vi "Test Pixy2 Functionality.vi"() -> ()   [LabVIEW 2018]
uses:
  source/library/Types/Intersection.ctl
  source/library/Types/Vector.ctl
  <vilib>/Rock Robotics/WPI/SerialPort/WPI_SerialPort.ctl
  source/library/Interface/Pixy Com.lvclass
  source/deviceSupport/FRC/I2C/RoboRIO I2C.lvclass
  <vilib>/Rock Robotics/SystemInterfaces/i2clib/i2c_bus.ctl
  source/library/Pixy2.lvlib
  <vilib>/Rock Robotics/SystemInterfaces/spilib/spi_bus.ctl
  source/deviceSupport/FRC/SPI/RoboRIO SPI.lvclass
  source/deviceSupport/FRC/UART/RoboRIO UART.lvclass
panel:
  out "vectors":T1[](array[typedef])
  out "intersections":T2[](array[typedef])
  out "view":picture
  in  "Stop Button":bool
  in  "message":enum32{"RGB", "Lamp", "Blocks", "Lines"}(tab)
  in  "color":cluster{"r":u8, "g":u8, "b":u8}
  in  "lamp enable":cluster{"upper":bool, "lower":bool}
  in  "signature map":u8=255 format="%.0x"
  in  "max blocks":u8=255
  in  "features":enum16{"Main Features", "All Features"}(ring)
  in  "feature map":u8=7 format="%.0x"
  out "error out":errorcluster
  in  "send":bool
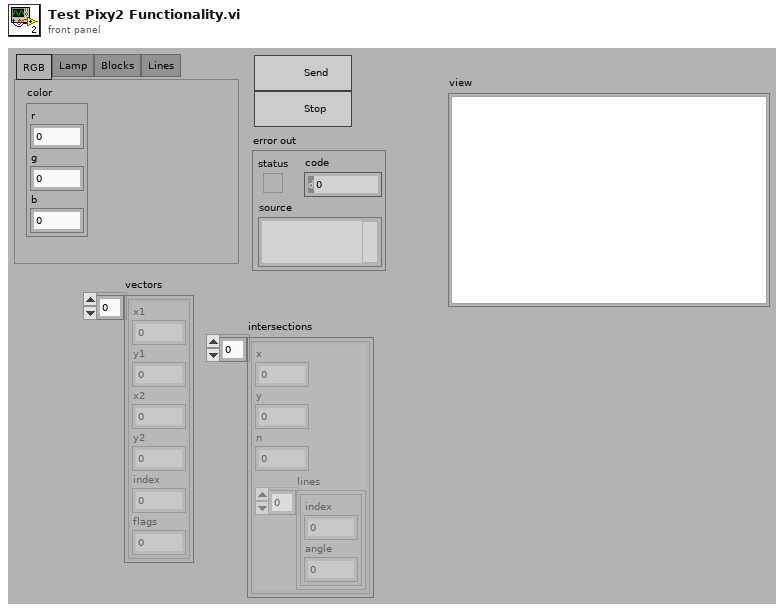
[diagram p1: front panel]
types:
  T1 = typedef "Pixy2.lvlib/Vector.ctl" = cluster{"x1":u8, "y1":u8, "x2":u8, "y2":u8, "index":u8, "flags":u8}
  T2 = typedef "Pixy2.lvlib/Intersection.ctl" = cluster{"x":u8, "y":u8, "n":u8, "lines":cluster{"index":u8, "angle":i16}[]}
  T3 = typedef "i2c_bus.ctl" = enum16{"I2C On-Board", "I2C MXP", "Invalid"}
  T4 = typedef "spi_bus.ctl" = enum16{"SPI On-Board, CS0", "SPI On-Board, CS1", "SPI On-Board, CS2", "SPI On-Board, CS3", "SPI MXP", "Invalid"}
  T5 = typedef "WPI_SerialPort.ctl" = enum16{"Onboard RS-232", "MXP TTL", "USB 1", "USB 2"}
  T6 = typedef "Pixy2.lvlib/Block.ctl" = cluster{"signature":u16, "x":u16, "y":u16, "width":u16, "height":u16, "angle":i16, "index":u8, "age":u8}
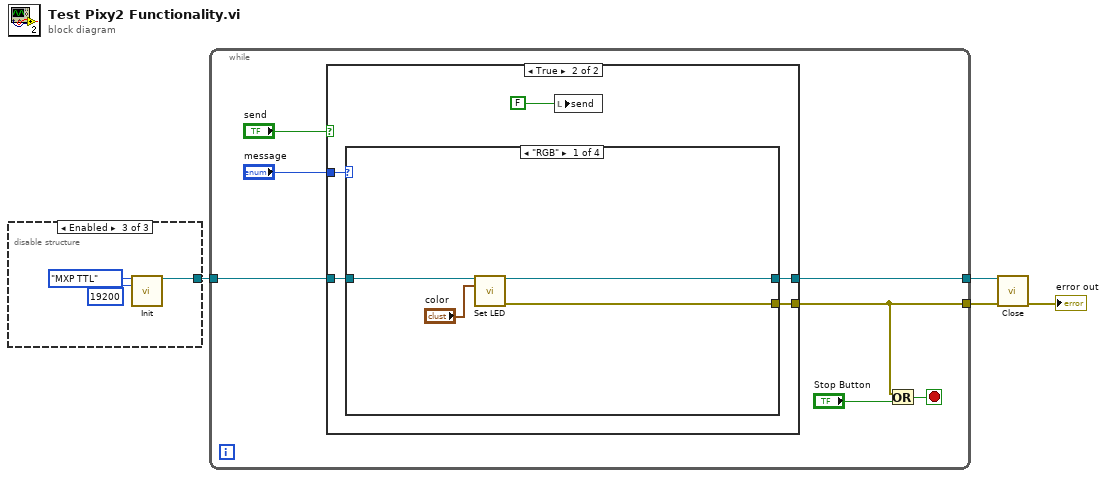
[diagram p0: block diagram]
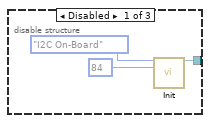
[diagram p2: hidden frame]
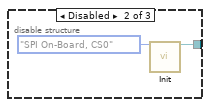
[diagram p3: hidden frame]
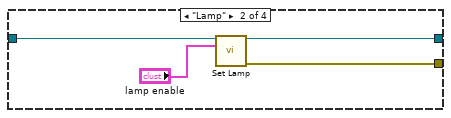
[diagram p5: hidden frame]
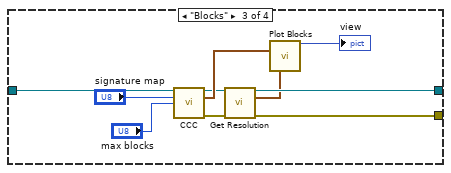
[diagram p6: hidden frame]
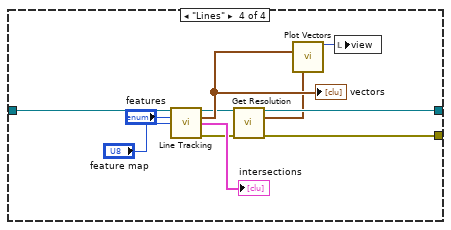
[diagram p7: hidden frame]
diagram:
  n1 = disable-structure shown="Enabled" {
    disable-tunnel: [w7 w9 w12] -> w4
    frame Disabled {
      n2 = call "Init.vi"("I2C Bus"=i2c_bus."I2C On-Board", "Device Address"=u8 84) -> ("comm interface out"=w7:refnum<class "Pixy Com.lvclass">)  [unwired: 12 in, 1 out]
    }
    frame Disabled {
      n3 = call "Init.vi"("SPI Bus"=spi_bus."SPI On-Board, CS0") -> ("comm interface out"=w9:refnum<class "Pixy Com.lvclass">)  [unwired: 13 in, 1 out]
    }
    frame Enabled {
      n4 = call "Init.vi"("serial port"=WPI_SerialPort."MXP TTL", "baud rate"=u32 19200) -> ("comm interface out"=w12:refnum<class "Pixy Com.lvclass">)  [unwired: 12 in, 1 out]
    }
  }
  n5 = while {
    tunnel: w4 -> [w18]
    tunnel: [w16] -> w3
    tunnel: [w17] -> w2
    stop <- w15 stop-if-true
    n6 = case shown="True" "send" {
      tunnel: w18 -> [w20 w24]
      tunnel: [_ w22] -> w16
      tunnel: [w20 w23] -> w17
      tunnel: "message" -> [_ w21]
      frame False {
      }
      frame True {
        n7 = case shown="\"RGB\"" w21 {
          tunnel: w24 -> [w29 w33 w43 w54]
          tunnel: [w28 w32 w35 w46] -> w23
          tunnel: [w27 w30 w36 w45] -> w22
          frame "RGB" {
            n8 = call "Set LED.vi"("comm interface in"=w29, "color"="color") -> ("comm interface out"=w28:refnum<class "Pixy Com.lvclass">, "error out"=w27:errorcluster)  [unwired: 12 in]
          }
          frame "Lamp" {
            n9 = call "Set Lamp.vi"("comm interface in"=w33, "lamp enable"="lamp enable") -> ("comm interface out"=w32:refnum<class "Pixy Com.lvclass">, "error out"=w30:errorcluster)  [unwired: 12 in]
          }
          frame "Blocks" {
            n10 = call "CCC.vi"("comm interface in"=w43, "signature map"="signature map", "max blocks"="max blocks") -> ("comm interface out"=w38:refnum<class "Pixy Com.lvclass">, "blocks"=w40:T6[], "error out"=w37:errorcluster)  [unwired: 10 in]
            n11 = call "Get Resolution.vi"("comm interface in"=w38, "error in"=w37) -> ("comm interface out"=w35:refnum<class "Pixy Com.lvclass">, "resolution"=w34:cluster{"width":u16, "height":u16}, "error out"=w36:errorcluster)  [unwired: 11 in]
            n12 = call "Plot Blocks.vi"("blocks"=w40, "pixy resolution"=w34) -> ("picture out"=→"view":picture)  [unwired: 13 in]
          }
          frame "Lines" {
            n13 = call "Line Tracking.vi"("comm interface in"=w54, "features"="features", "feature map"="feature map") -> ("comm interface out"=w48:refnum<class "Pixy Com.lvclass">, "vectors"=w51:T1[], "intersections"=→"intersections":T2[], "error out"=w47:errorcluster)  [unwired: 8 in, 1 out]
            "vectors" <- w51
            n14 = call "Get Resolution.vi"("comm interface in"=w48, "error in"=w47) -> ("comm interface out"=w46:refnum<class "Pixy Com.lvclass">, "resolution"=w44:cluster{"width":u16, "height":u16}, "error out"=w45:errorcluster)  [unwired: 11 in]
            n15 = call "Plot Vectors.vi"("vectors"=w51, "pixy resolution"=w44) -> ("picture out"=w50:picture)  [unwired: 13 in]
            n16 = local write "view"(w50) -> ()
          }
        }
        n17 = local write "send"(FALSE ("send button")) -> ()
      }
    }
    n18 = Or(x=w16, y="Stop Button") -> (x .or. y?=w15:bool)
  }
  n19 = call-dynamic "Close.vi"("comm interface in"=w2, "error in"=w3) -> ("error out"=→"error out":errorcluster)  [unwired: 13 in]
